vi "FindLowerCornerConnectorPaneTerminals.vi"(8 "error in (no error)":errorcluster, 11 "VI reference":refnum<vi>) -> (0 "error out":errorcluster, 1 "Bottom right index":u32, 2 "Bottom left index":u32, 3 "VI reference (dup)":refnum<vi>)   [LabVIEW 2017, in "ErrorStructureDrawer.lvlib"]
doc: "Returns the indices of the bottom-left and bottom-right connector pane terminals of the specified VI."
uses:
  ErrorStructureDrawer.lvlib
  Controls/ConnectorPaneTerminalInfo.ctl
  <vilib>/Utility/miscctls.llb/LVRectTypeDef.ctl
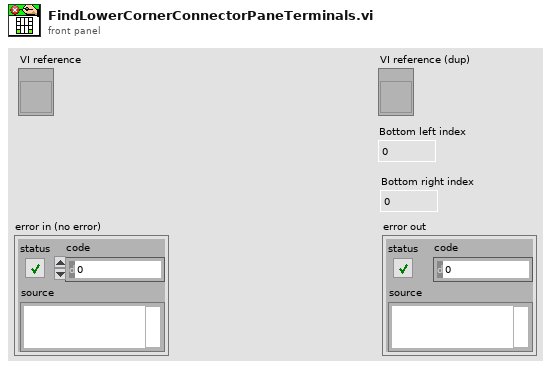
[diagram p1: front panel]
types:
  T1 = typedef "ErrorStructureDrawer.lvlib/ConnectorPaneTerminalInfo.ctl" = cluster{"Index":u32, "Position":T2}
  T2 = typedef "LVRectTypeDef.ctl" = cluster{"Left":i16, "Top":i16, "Right":i16, "Bottom":i16}
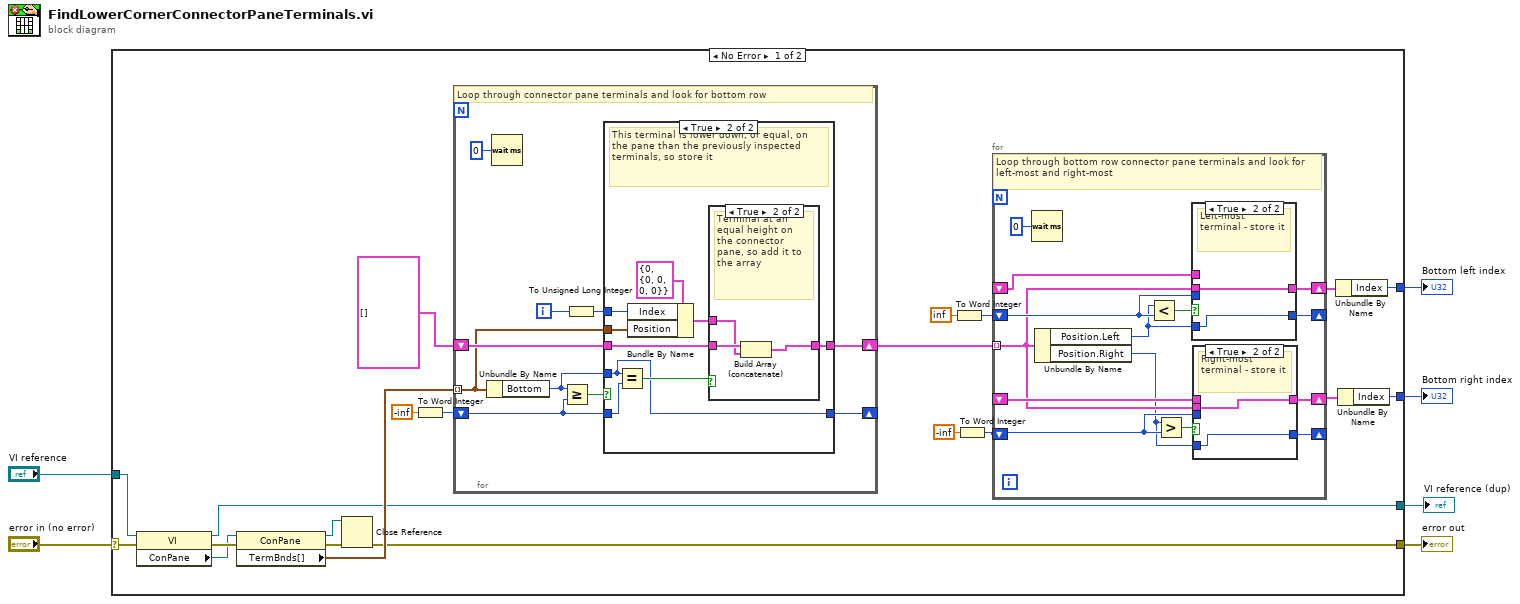
[diagram p0: block diagram]
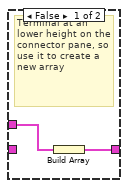
[diagram p3: hidden frame]
diagram:
  n1 = case shown="No Error" "error in (no error)" {
    selector: "error in (no error)" -> [w9 w77]
    tunnel: [w16 _] -> w6
    tunnel: [w15 _] -> w5
    tunnel: "VI reference" -> [w11 w76]
    tunnel: [w10 w77] -> w3
    tunnel: [w8 w76] -> w1
    frame No Error {
      n2 = property class="VI"(reference=w11, error in=w9) -> (reference out=w8:refnum<vi>, error out=w27:errorcluster, "ConPane"=w23:refnum<vi>)
      n3 = property class="ConPane"(reference=w23, error in=w27) -> (reference out=w12:refnum<vi>, error out=w13:errorcluster, "TermBnds[]"=w26:T2[])
      n4 = Close Reference(reference=w12, error in (no error)=w13) -> (error out=w10:errorcluster)
      n5 = To Word Integer(number=-inf) -> (16bit integer=w24:i16)
      n6 = for {
        tunnel: w26 -> [w31] mode=indexing
        shift-right: [w34] -> w22
        shift-left: T1[] [] -> [w33]
        shift-right: [w32] -> _
        shift-left: w24 -> [w35]
        i -> [w29]
        # "Loop through connector pane terminals and look for bottom row"
        n7 = Unbundle By Name(w31) -> ("Bottom"=w36:i16)
        n8 = Wait (ms)(milliseconds to wait=u32 0) -> ()  [unwired: 1 out]
        n9 = Greater Or Equal?(x=w36, y=w35) -> (x >= y?=w37:bool)
        n10 = To Unsigned Long Integer(number=w29) -> (unsigned 32bit integer=w30:u32)
        n11 = case shown="True" w37 {
          tunnel: w36 -> [_ w44]
          tunnel: w35 -> [w38 w45]
          tunnel: [w39 w47] -> w34
          tunnel: w33 -> [w39 w46]
          tunnel: [w38 w44] -> w32
          tunnel: w31 -> [_ w42]
          tunnel: w30 -> [_ w43]
          frame False {
            # "This terminal is higher up on the pane than the previously inspected terminals, so ignore it"
          }
          frame True {
            # "This terminal is lower down, or equal, on the pane than the previously inspected terminals, so store it"
            n12 = Equal?(x=w44, y=w45) -> (x = y?=w48:bool)
            n13 = Bundle By Name(cluster=T1 {"Index"=0, "Position"={"Left"=0, "Top"=0, "Right"=0, "Bottom"=0}} ("Connector pane terminal info"), "Index"=w43, "Position"=w42) -> (w41:T1)
            n14 = case shown="True" w48 {
              tunnel: [w50 w53] -> w47
              tunnel: w46 -> [_ w52]
              tunnel: w41 -> [w49 w51]
              frame False {
                # "Terminal at an lower height on the connector pane, so use it to create a new array"
                n15 = Build Array(w49) -> (w50:T1[])
              }
              frame True {
                # "Terminal at an equal height on the connector pane, so add it to the array"
                n16 = Build Array (concatenate)(w52, w51) -> (w53:T1[])
              }
            }
          }
        }
      }
      n17 = To Word Integer(number=inf) -> (16bit integer=w19:i16)
      n18 = To Word Integer(number=-inf) -> (16bit integer=w18:i16)
      n19 = for {
        tunnel: w22 -> [w57] mode=indexing
        shift-right: [w64] -> _
        shift-left: w19 -> [w63]
        shift-right: [w62] -> _
        shift-left: w18 -> [w60]
        shift-right: [w66] -> w17
        shift-left: _ -> [w65]
        shift-right: [w59] -> w14
        shift-left: _ -> [w58]
        # "Loop through bottom row connector pane terminals and look for left-most and right-most"
        n20 = Wait (ms)(milliseconds to wait=u32 0) -> ()  [unwired: 1 out]
        n21 = Unbundle By Name(w57) -> ("Position.Left"=w55:i16, "Position.Right"=w56:i16)
        n22 = Less?(x=w55, y=w63) -> (x < y?=w67:bool)
        n23 = Greater?(x=w56, y=w60) -> (0:w61:bool)
        n24 = case shown="True" w67 {
          tunnel: w57 -> [_ w75]
          tunnel: [w73 w75] -> w66
          tunnel: w65 -> [w73 _]
          tunnel: w55 -> [_ w74]
          tunnel: [w72 w74] -> w64
          tunnel: w63 -> [w72 _]
          frame False {
            # "Not left-most terminal - do nothing"
          }
          frame True {
            # "Left-most terminal - store it"
          }
        }
        n25 = case shown="True" w61 {
          tunnel: w57 -> [_ w71]
          tunnel: [w69 w71] -> w59
          tunnel: w58 -> [w69 _]
          tunnel: w56 -> [_ w70]
          tunnel: [w68 w70] -> w62
          tunnel: w60 -> [w68 _]
          frame False {
            # "Not right-most terminal - do nothing"
          }
          frame True {
            # "Right-most terminal - store it"
          }
        }
      }
      n26 = Unbundle By Name(w17) -> ("Index"=w16:u32)
      n27 = Unbundle By Name(w14) -> ("Index"=w15:u32)
    }
    frame Error {
    }
  }
  "Bottom left index" <- w6
  "Bottom right index" <- w5
  "error out" <- w3
  "VI reference (dup)" <- w1
